vi "e^2.vi"(4 "Parametry Ziemi":T1={"a - półoś duża"=6378137.0, "b - półoś mała"=6356752.3141999999998} {"b - półoś mała" format="%_20f"; "a - półoś duża" format="%_20g"}) -> (1 "e^2":ext=6378137.0 format="%_20g")   [LabVIEW 2015, in "Biblioteka moduł map v3.lvlib" / "Konwersja wsp.lvlib" / "UTM.lvlib"]
uses:
  UTM.lvlib
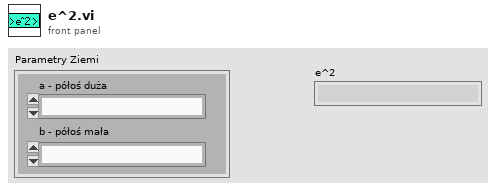
[diagram p1: front panel]
types:
  T1 = cluster{"a - półoś duża":ext, "b - półoś mała":ext}
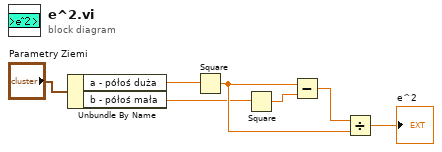
[diagram p0: block diagram]
diagram:
  n1 = Unbundle By Name("Parametry Ziemi") -> ("a - półoś duża"=w3:ext, "b - półoś mała"=w2:ext)
  n2 = Square(x=w3) -> (x^2=w6:ext)
  n3 = Square(x=w2) -> (x^2=w5:ext)
  n4 = Subtract(x=w6, y=w5) -> (x-y=w7:ext)
  n5 = Divide(x=w7, y=w6) -> (x/y=→"e^2":ext)
